vi "段内码.vi"(9 "参考电压（V）":dbl, 10 "段落位置":dbl, 11 "信号电压":dbl) -> (3 "段内码":ext)   [LabVIEW 2018]
panel:
  # "输入：段落位置n，参考电压Vref，信号电压\n输出：对应的段内码（十进制）"
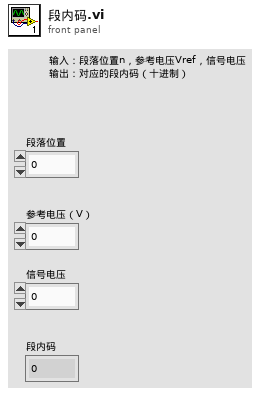
[diagram p1: front panel]
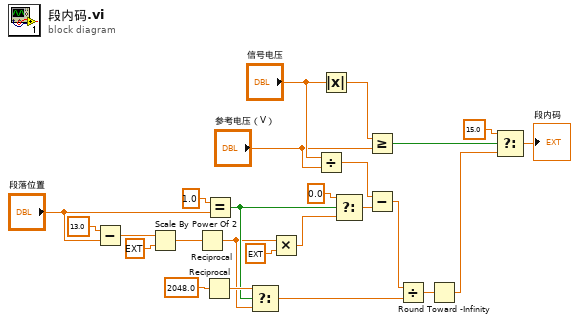
[diagram p0: block diagram]
diagram:
  n1 = Subtract(x=13.0, y="段落位置") -> (x-y=w24:dbl)
  n2 = Scale By Power Of 2(n=w24, x=ext 1.0) -> (x*2^n=w22:ext)
  n3 = Reciprocal(x=w22) -> (1/x=w13:ext)
  n4 = Reciprocal(x=2048.0) -> (1/x=w19:dbl)
  n5 = Equal?(x=1.0, y="段落位置") -> (x = y?=w17:bool)
  n6 = Select(t=w19, s=w17, f=w13) -> (s? t:f=w9:ext)
  n7 = Multiply(x=w13, y=ext 16.0) -> (x*y=w12:ext)
  n8 = Divide(x="信号电压", y="参考电压（V）") -> (x/y=w11:dbl)
  n9 = Absolute Value(x="信号电压") -> (abs(x)=w3:dbl)
  n10 = Select(t=0.0, s=w17, f=w12) -> (s? t:f=w15:ext)
  n11 = Greater Or Equal?(x=w3, y="参考电压（V）") -> (x >= y?=w1:bool)
  n12 = Subtract(x=w11, y=w15) -> (x-y=w10:ext)
  n13 = Divide(x=w10, y=w9) -> (x/y=w8:ext)
  n14 = Round Toward -Infinity(1:w8) -> (0:w5:ext)
  n15 = Select(t=15.0, s=w1, f=w5) -> (s? t:f=→"段内码":ext)
